vi "INI-RWOneVar-EnFlo.vi"(6 "Mode":enum16{"Read", "Write"}(ring), 7 "section":string, 9 "controlRefIn":refnum<vi>, 11 "INIfileRefIn":T3) -> (0 "error out":errorcluster, 3 "INIfileRefOut":T3)   [LabVIEW 2022 SP3]
uses:
  <vilib>/Utility/config.llb/Config Data RefNum.ctl
  Anemometry Sub Vis/File/INIfiles/dataTypeForINIfile-EnFlo.ctl
  <vilib>/Utility/Data Type/Type Definitions/Data Type.ctl
  Anemometry Sub Vis/Globals/Constants_global.vi
  <vilib>/Utility/config.llb/Read Key (Boolean).vi
  <vilib>/Utility/config.llb/Read Key (U32).vi
  <vilib>/Utility/config.llb/Read Key (I32).vi
  <vilib>/Utility/config.llb/Read Key (Double).vi
  <vilib>/Utility/config.llb/Read Key (Path).vi
  <vilib>/Utility/config.llb/Read Key (String).vi
  <vilib>/Utility/config.llb/Write Key (Boolean).vi
  <vilib>/Utility/config.llb/Write Key (U32).vi
  <vilib>/Utility/config.llb/Write Key (I32).vi
  <vilib>/Utility/config.llb/Write Key (Double).vi
  <vilib>/Utility/config.llb/Write Key (Path).vi
  <vilib>/Utility/config.llb/Write Key (String).vi
  <vilib>/Utility/Data Type/NI_Data Type.lvlib
  <vilib>/Utility/config.llb/NI_LVConfig.lvlib
panel:
  out "badRefOut":bool
  out "type":T1
  out "storeAs":T2
  out "badRefIn":bool
  out "Label.Text":string
  out "Value":variant
  # "Makes best-effort to save or restore the value of the referred control"
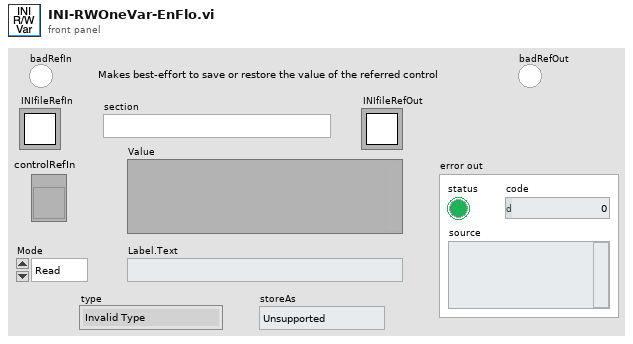
[diagram p1: front panel]
types:
  T1 = typedef "NI_Data Type.lvlib/Data Type.ctl" = enum8{"Invalid Type", "Void", "I8", "I16", "I32", "I64", "U8", "U16", "U32", "U64", "Single Float", "Double Float", "Extended Float", "Single Complex", "Double Complex", "Extended Complex", "Enum U8", "Enum U16", "Enum U32", "Enum U64", "Single Float With Unit", "Double Float With Unit", "Extended Float With Unit", "Single Complex with Unit", "Double Complex with Unit", "Extended Complex with Unit", "Boolean", "String", "Path", "Picture", "Tag", "Array", "Cluster", "Variant", "LV Variant", "Waveform", "Timestamp", "Digital Waveform", "Digital Data", "ExpressData", "Refnum", "External Data", "VI", "Poly VI", "LabVIEW Class Instance", "Fixed Point", "Set Collection", "Map Collection"}
  T2 = typedef "dataTypeForINIfile-EnFlo.ctl" = enum16{"Unsupported", "Boolean", "U32", "I32", "Double", "Path", "String", "Special"}
  T3 = typedef "NI_LVConfig.lvlib/Config Data RefNum.ctl" = refnum<k1>
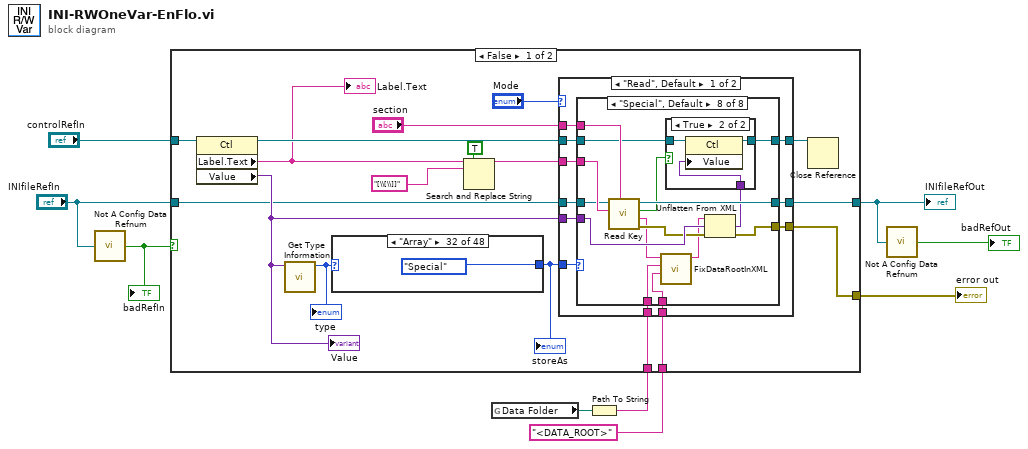
[diagram p0: block diagram]
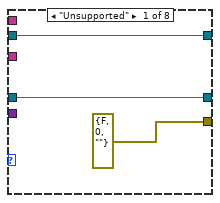
[diagram p2: hidden frame]
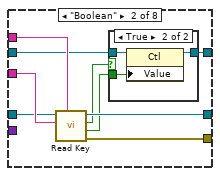
[diagram p3: hidden frame]
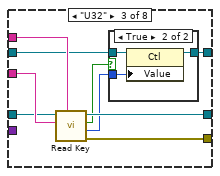
[diagram p5: hidden frame]
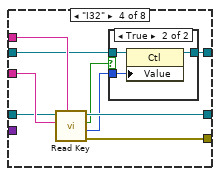
[diagram p7: hidden frame]
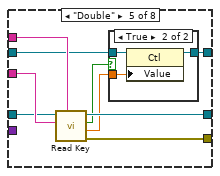
[diagram p9: hidden frame]
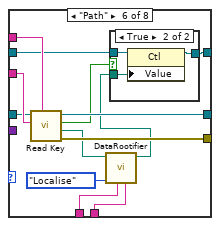
[diagram p11: hidden frame]
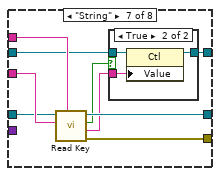
[diagram p13: hidden frame]
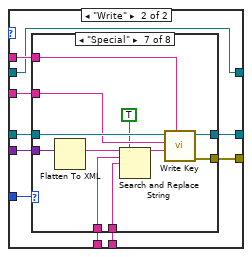
[diagram p16: hidden frame]
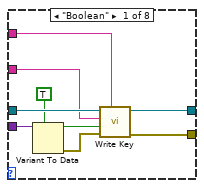
[diagram p17: hidden frame]
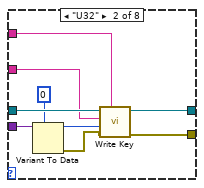
[diagram p18: hidden frame]
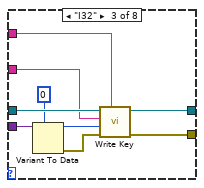
[diagram p19: hidden frame]
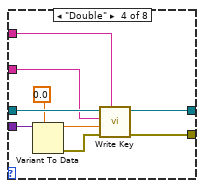
[diagram p20: hidden frame]
diagram:
  n1 = call <vilib>:"Not A Config Data Refnum.vi"("refnum"="INIfileRefIn") -> ("not a config data refnum"=w6:bool)
  "badRefIn" <- w6
  n2 = global read "Constants_global.vi" "Data Folder"() -> (w3:path)
  n3 = Path To String(path=w3) -> (string=w2:string)
  n4 = case shown="False" w6 {
    tunnel: "controlRefIn" -> [w19 _]
    tunnel: [w18 errorcluster {"status"=FALSE, "code"=0, "source"=""} ("error out")] -> w8
    tunnel: [w17 w276] -> w5
    tunnel: "INIfileRefIn" -> [w16 w276]
    tunnel: w2 -> [w11 _]
    tunnel: "<DATA_ROOT>" ("regular expression") -> [w10 _]
    frame False {
      n5 = property class="Ctl"(reference=w19) -> (reference out=w23:refnum<vi>, "Label.Text"=w14:string, "Value"=w21:variant)  [unwired: 1 in, 1 out]
      "Value" <- w21
      "Label.Text" <- w14
      n6 = call <vilib>:"Get Type Information.vi"("variant"=w21) -> ("type"=w25:T1)  [unwired: 6 in, 4 out]
      "type" <- w25
      n7 = case shown="\"Array\"" w25 {
        tunnel: [dataTypeForINIfile-EnFlo."Unsupported" dataTypeForINIfile-EnFlo."Unsupported" dataTypeForINIfile-EnFlo."I32" dataTypeForINIfile-EnFlo."I32" dataTypeForINIfile-EnFlo."I32" dataTypeForINIfile-EnFlo."Special" dataTypeForINIfile-EnFlo."U32" dataTypeForINIfile-EnFlo."U32" dataTypeForINIfile-EnFlo."U32" dataTypeForINIfile-EnFlo."Special" dataTypeForINIfile-EnFlo."Double" dataTypeForINIfile-EnFlo."Double" dataTypeForINIfile-EnFlo."Special" dataTypeForINIfile-EnFlo."Special" dataTypeForINIfile-EnFlo."Special" dataTypeForINIfile-EnFlo."Special" dataTypeForINIfile-EnFlo."U32" dataTypeForINIfile-EnFlo."U32" dataTypeForINIfile-EnFlo."U32" dataTypeForINIfile-EnFlo."Special" dataTypeForINIfile-EnFlo."Special" dataTypeForINIfile-EnFlo."Special" dataTypeForINIfile-EnFlo."Special" dataTypeForINIfile-EnFlo."Special" dataTypeForINIfile-EnFlo."Special" dataTypeForINIfile-EnFlo."Special" dataTypeForINIfile-EnFlo."Boolean" dataTypeForINIfile-EnFlo."String" dataTypeForINIfile-EnFlo."Path" dataTypeForINIfile-EnFlo."Special" dataTypeForINIfile-EnFlo."Special" dataTypeForINIfile-EnFlo."Special" dataTypeForINIfile-EnFlo."Special" dataTypeForINIfile-EnFlo."Special" dataTypeForINIfile-EnFlo."Unsupported" dataTypeForINIfile-EnFlo."Special" dataTypeForINIfile-EnFlo."Double" dataTypeForINIfile-EnFlo."Special" dataTypeForINIfile-EnFlo."Special" dataTypeForINIfile-EnFlo."Unsupported" dataTypeForINIfile-EnFlo."Unsupported" dataTypeForINIfile-EnFlo."Unsupported" dataTypeForINIfile-EnFlo."Unsupported" dataTypeForINIfile-EnFlo."Unsupported" dataTypeForINIfile-EnFlo."Unsupported" dataTypeForINIfile-EnFlo."Special" dataTypeForINIfile-EnFlo."Special" dataTypeForINIfile-EnFlo."Special"] -> w20
        frame "Invalid Type", Default {
        }
        frame "Void" {
        }
        frame "I8" {
        }
        frame "I16" {
        }
        frame "I32" {
        }
        frame "I64" {
        }
        frame "U8" {
        }
        frame "U16" {
        }
        frame "U32" {
        }
        frame "U64" {
        }
        frame "Single Float" {
        }
        frame "Double Float" {
        }
        frame "Extended Float" {
        }
        frame "Single Complex" {
        }
        frame "Double Complex" {
        }
        frame "Extended Complex" {
        }
        frame "Enum U8" {
        }
        frame "Enum U16" {
        }
        frame "Enum U32" {
        }
        frame "Enum U64" {
        }
        frame "Single Float With Unit" {
        }
        frame "Double Float With Unit" {
        }
        frame "Extended Float With Unit" {
        }
        frame "Single Complex with Unit" {
        }
        frame "Double Complex with Unit" {
        }
        frame "Extended Complex with Unit" {
        }
        frame "Boolean" {
        }
        frame "String" {
        }
        frame "Path" {
        }
        frame "Picture" {
        }
        frame "Tag" {
        }
        frame "Array" {
        }
        frame "Cluster" {
        }
        frame "Variant" {
        }
        frame "LV Variant" {
        }
        frame "Waveform" {
        }
        frame "Timestamp" {
        }
        frame "Digital Waveform" {
        }
        frame "Digital Data" {
        }
        frame "ExpressData" {
        }
        frame "Refnum" {
        }
        frame "External Data" {
        }
        frame "VI" {
        }
        frame "Poly VI" {
        }
        frame "LabVIEW Class Instance" {
        }
        frame "Fixed Point" {
        }
        frame "Set Collection" {
        }
        frame "Map Collection" {
        }
      }
      "storeAs" <- w20
      n8 = Search and Replace String(replace all?=TRUE ("replace all? (F)"), input string=w14, search string="[\\[\\]]") -> (result string=w15:string)  [unwired: 5 in, 3 out]
      n9 = case shown="\"Read\", Default" "Mode" {
        tunnel: w20 -> [w37 w151]
        tunnel: w16 -> [w32 w150]
        tunnel: w15 -> [w36 w149]
        tunnel: w21 -> [w31 w148]
        tunnel: [w33 w147] -> w17
        tunnel: "section" -> [w35 w146]
        tunnel: w23 -> [w34 w145]
        tunnel: [w30 w145] -> w26
        tunnel: [w29 w144] -> w18
        tunnel: w11 -> [w27 w143]
        tunnel: w10 -> [w28 w142]
        frame "Read", Default {
          n10 = case shown="\"Special\", Default" w37 {
            tunnel: w35 -> [_ w49 w62 w75 w88 w105 w118 w137]
            tunnel: w36 -> [_ w48 w61 w74 w87 w104 w117 w136]
            tunnel: [w40 w47 w60 w73 w86 w103 w116 w135] -> w33
            tunnel: w34 -> [w39 w44 w57 w70 w83 w102 w113 w134]
            tunnel: w32 -> [w40 w46 w59 w72 w85 w101 w115 w133]
            tunnel: w31 -> [_ _ _ _ _ _ _ w130]
            tunnel: [w39 w45 w58 w71 w84 w100 w114 w131] -> w30
            tunnel: [errorcluster {"status"=FALSE, "code"=0, "source"=""} ("error out") w41 w54 w67 w80 w98 w110 w127] -> w29
            tunnel: w28 -> [_ _ _ _ _ w94 _ w126]
            tunnel: w27 -> [_ _ _ _ _ w93 _ w125]
            frame "Unsupported" {
            }
            frame "Boolean" {
              n11 = call-poly <vilib>:"Read Key.vi"("section"=w49, "key"=w48, "refnum"=w46) -> ("error out"=w41:errorcluster, "value"=w42:bool, "found?"=w43:bool, "refnum out"=w47:T3)  [unwired: 5 in]
              n12 = case shown="True" w43 {
                tunnel: w44 -> [w50 w53]
                tunnel: w42 -> [_ w52]
                tunnel: [w50 w51] -> w45
                frame False {
                }
                frame True {
                  n13 = property class="Ctl"(reference=w53, "Value"=w52) -> (reference out=w51:refnum<vi>)  [unwired: 1 in, 1 out]
                }
              }
            }
            frame "U32" {
              n14 = call-poly <vilib>:"Read Key.vi"("section"=w62, "key"=w61, "refnum"=w59) -> ("error out"=w54:errorcluster, "value"=w55:u32, "found?"=w56:bool, "refnum out"=w60:T3)  [unwired: 5 in]
              n15 = case shown="True" w56 {
                tunnel: w57 -> [w63 w66]
                tunnel: w55 -> [_ w65]
                tunnel: [w63 w64] -> w58
                frame False {
                }
                frame True {
                  n16 = property class="Ctl"(reference=w66, "Value"=w65) -> (reference out=w64:refnum<vi>)  [unwired: 1 in, 1 out]
                }
              }
            }
            frame "I32" {
              n17 = call-poly <vilib>:"Read Key.vi"("section"=w75, "key"=w74, "refnum"=w72) -> ("error out"=w67:errorcluster, "value"=w69:i32, "found?"=w68:bool, "refnum out"=w73:T3)  [unwired: 5 in]
              n18 = case shown="True" w68 {
                tunnel: [w76 w79] -> w71
                tunnel: w70 -> [w76 w78]
                tunnel: w69 -> [_ w77]
                frame False {
                }
                frame True {
                  n19 = property class="Ctl"(reference=w78, "Value"=w77) -> (reference out=w79:refnum<vi>)  [unwired: 1 in, 1 out]
                }
              }
            }
            frame "Double" {
              n20 = call-poly <vilib>:"Read Key.vi"("section"=w88, "key"=w87, "refnum"=w85) -> ("error out"=w80:errorcluster, "value"=w81:dbl, "found?"=w82:bool, "refnum out"=w86:T3)  [unwired: 5 in]
              n21 = case shown="True" w82 {
                tunnel: w83 -> [w89 w92]
                tunnel: w81 -> [_ w91]
                tunnel: [w89 w90] -> w84
                frame False {
                }
                frame True {
                  n22 = property class="Ctl"(reference=w92, "Value"=w91) -> (reference out=w90:refnum<vi>)  [unwired: 1 in, 1 out]
                }
              }
            }
            frame "Path" {
              n23 = call-poly <vilib>:"Read Key.vi"("section"=w105, "key"=w104, "refnum"=w101) -> ("error out"=w98:errorcluster, "value"=w97:path, "found?"=w99:bool, "refnum out"=w103:T3)  [unwired: 5 in]
              n24 = call "DataRootifier.vi"("pathPlaceholder"=w94, "replacePathPortion"=w93, "mode"=enum16{"Generalise", "Localise"}."Localise", "pathIn"=w97) -> ("pathOut"=w96:path)  [unwired: 7 in]
              n25 = case shown="True" w99 {
                tunnel: w102 -> [w106 w109]
                tunnel: w96 -> [_ w108]
                tunnel: [w106 w107] -> w100
                frame False {
                }
                frame True {
                  n26 = property class="Ctl"(reference=w109, "Value"=w108) -> (reference out=w107:refnum<vi>)  [unwired: 1 in, 1 out]
                }
              }
            }
            frame "String" {
              n27 = call-poly <vilib>:"Read Key.vi"("section"=w118, "key"=w117, "refnum"=w115) -> ("error out"=w110:errorcluster, "value"=w112:string, "found?"=w111:bool, "refnum out"=w116:T3)  [unwired: 5 in]
              n28 = case shown="True" w111 {
                tunnel: [w119 w122] -> w114
                tunnel: w113 -> [w119 w121]
                tunnel: w112 -> [_ w120]
                frame False {
                }
                frame True {
                  n29 = property class="Ctl"(reference=w121, "Value"=w120) -> (reference out=w122:refnum<vi>)  [unwired: 1 in, 1 out]
                }
              }
            }
            frame "Special", Default {
              n30 = call-poly <vilib>:"Read Key.vi"("section"=w137, "key"=w136, "refnum"=w133) -> ("error out"=w128:errorcluster, "value"=w124:string, "found?"=w129:bool, "refnum out"=w135:T3)  [unwired: 5 in]
              n31 = call "FixDataRootInXML.vi"("pathPlaceholderString"=w126, "replacementPath"=w125, "XMLstringIn"=w124) -> ("XMLstringOut"=w123:string)  [unwired: 8 in]
              n32 = Unflatten From XML(xml string=w123, type=w130, error in (no error)=w128) -> (value=w132:variant, error out=w127:errorcluster)
              n33 = case shown="True" w129 {
                tunnel: w134 -> [w138 w141]
                tunnel: w132 -> [_ w140]
                tunnel: [w138 w139] -> w131
                frame False {
                }
                frame True {
                  n34 = property class="Ctl"(reference=w141, "Value"=w140) -> (reference out=w139:refnum<vi>)  [unwired: 1 in, 1 out]
                }
              }
            }
          }
        }
        frame "Write" {
          n35 = case shown="\"Special\"" w151 {
            tunnel: w150 -> [w160 w169 w178 w187 w200 w209 w220 w226]
            tunnel: w146 -> [w159 w168 w177 w186 w199 w208 w219 w225]
            tunnel: w149 -> [w158 w167 w176 w185 w198 w207 w218 w224]
            tunnel: w148 -> [w157 w166 w175 w184 w197 w206 w216 _]
            tunnel: [w154 w163 w172 w181 w195 w205 w217 w223] -> w147
            tunnel: [w152 w161 w170 w179 w193 w203 w215 w221] -> w144
            tunnel: w143 -> [_ _ _ _ w190 _ w211 _]
            tunnel: w142 -> [_ _ _ _ w189 _ w210 _]
            frame "Boolean" {
              n36 = Variant To Data(type=TRUE, Variant=w157) -> (data=w156:bool, error out=w153:errorcluster)  [unwired: 1 in]
              n37 = call-poly <vilib>:"Write Key.vi"("section"=w159, "error in (no error)"=w153, "value"=w156, "key"=w158, "refnum"=w160) -> ("error out"=w152:errorcluster, "refnum out"=w154:T3)  [unwired: 4 in, 1 out]
            }
            frame "U32" {
              n38 = Variant To Data(type=u32 0, Variant=w166) -> (data=w165:u32, error out=w162:errorcluster)  [unwired: 1 in]
              n39 = call-poly <vilib>:"Write Key.vi"("section"=w168, "error in (no error)"=w162, "value"=w165, "key"=w167, "refnum"=w169) -> ("error out"=w161:errorcluster, "refnum out"=w163:T3)  [unwired: 4 in, 1 out]
            }
            frame "I32" {
              n40 = Variant To Data(type=0, Variant=w175) -> (data=w174:i32, error out=w171:errorcluster)  [unwired: 1 in]
              n41 = call-poly <vilib>:"Write Key.vi"("section"=w177, "error in (no error)"=w171, "value"=w174, "key"=w176, "refnum"=w178) -> ("error out"=w170:errorcluster, "refnum out"=w172:T3)  [unwired: 4 in, 1 out]
            }
            frame "Double" {
              n42 = Variant To Data(type=0.0, Variant=w184) -> (data=w183:dbl, error out=w180:errorcluster)  [unwired: 1 in]
              n43 = call-poly <vilib>:"Write Key.vi"("section"=w186, "error in (no error)"=w180, "value"=w183, "key"=w185, "refnum"=w187) -> ("error out"=w179:errorcluster, "refnum out"=w181:T3)  [unwired: 4 in, 1 out]
            }
            frame "Path" {
              n44 = Variant To Data(type=path "", Variant=w197) -> (data=w192:path, error out=w194:errorcluster)  [unwired: 1 in]
              n45 = call "DataRootifier.vi"("pathPlaceholder"=w189, "replacePathPortion"=w190, "mode"=enum16{"Generalise", "Localise"}."Generalise", "pathIn"=w192) -> ("pathOut"=w191:path)  [unwired: 7 in]
              n46 = call-poly <vilib>:"Write Key.vi"("section"=w199, "error in (no error)"=w194, "value"=w191, "key"=w198, "refnum"=w200) -> ("error out"=w193:errorcluster, "refnum out"=w195:T3)  [unwired: 4 in, 1 out]
            }
            frame "String" {
              n47 = Variant To Data(type="", Variant=w206) -> (data=w201:string, error out=w204:errorcluster)  [unwired: 1 in]
              n48 = call-poly <vilib>:"Write Key.vi"("section"=w208, "error in (no error)"=w204, "value"=w201, "key"=w207, "refnum"=w209) -> ("error out"=w203:errorcluster, "refnum out"=w205:T3)  [unwired: 4 in, 1 out]
            }
            frame "Special" {
              n49 = Flatten To XML(6:w216) -> (2:w214:string)
              n50 = Search and Replace String(replace all?=TRUE ("replace all? (F)"), input string=w214, search string=w211, replace string=w210) -> (result string=w213:string)  [unwired: 4 in, 3 out]
              n51 = call-poly <vilib>:"Write Key.vi"("section"=w219, "value"=w213, "key"=w218, "refnum"=w220) -> ("error out"=w215:errorcluster, "refnum out"=w217:T3)  [unwired: 5 in, 1 out]
            }
            frame "Unsupported", Default {
              n52 = call-poly <vilib>:"Write Key.vi"("section"=w225, "value"="Sorry can't save this type", "key"=w224, "refnum"=w226) -> ("error out"=w221:errorcluster, "refnum out"=w223:T3)  [unwired: 5 in, 1 out]
            }
          }
        }
      }
      n53 = Close Reference(reference=w26) -> ()  [unwired: 1 in, 1 out]
    }
    frame True {
    }
  }
  "INIfileRefOut" <- w5
  "error out" <- w8
  n54 = call <vilib>:"Not A Config Data Refnum.vi"("refnum"=w5) -> ("not a config data refnum"=→"badRefOut":bool)
